vi "Apply.vi"(9 "Environment":T3, 10 "arguments":T1[](array[typedef]), 11 "function":T1) -> ()   [LabVIEW 2021]
uses:
  Expression.ctl
  ExpressionType.ctl
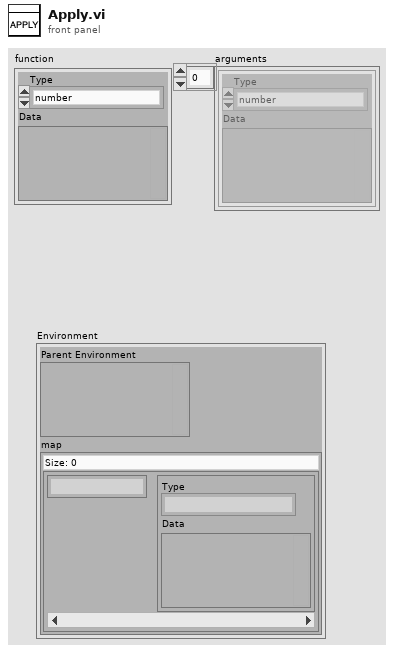
[diagram p1: front panel]
types:
  T1 = typedef "Expression.ctl" = cluster{"Type":T2, "Data":variant}
  T2 = typedef "ExpressionType.ctl" = enum16{"number", "string", "symbol", "primitive", "list", "closure", "macro", "nil", "error"}
  T3 = cluster{"Parent Environment":variant, "map":map{string, T1}}
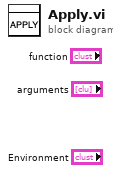
[diagram p0: block diagram]
diagram:
